vi "Task Map To Items.vi"   [LabVIEW 2024]
uses:
  Composite ID-Map Task.lvclass
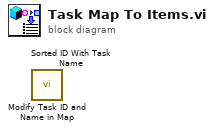
[diagram p0: block diagram]
diagram:
  n1 = call "Modify Task ID and Name in Map.vi"() -> ()  [unwired: 10 in, 2 out]
  n2 = call "Sorted ID With Task Name.vi"() -> ()  [unwired: 9 in, 3 out]
